vi "GIF.Write.Pack.Data.NormalizeImage__ogtk.vi"(9 "bottom":i16, 10 "right":i16, 11 "ImageIn":u8[](array[numeric])) -> (3 "ImageOut":u8[](array[numeric]))   [LabVIEW 2014]
panel:
  # "GIF.Write.Pack.Data.NormalizeImage.vi\n\nRemoves extra row padding-bytes.\n\nPlease visit http://www.OpenG.org to learn about the\nOpen Source LabVIEW software movement.\n\nNOTICE -- YOU MUST LEAVE THIS NOTICE IN PLACE.  PER THE TERMS OF THE LICENSE BELOW, YOU MAY SUBLICENSE THIS SOFTWARE \nIN ANY WAY THAT DOES NOT CONFLICT WITH THIS LICENSE.\n\n### BSD License (http://www.opensource.org/licenses/bsd-license.php) Begin ###\n \nCopyright (c) 2007, Bill Clench <bclench@yahoo.com>\n\nAll rights reserved.\n\nRedistribution and use in source and binary forms, with or without modification, are permitted provided that the following conditions are met:\n\n    * Redistributions of source code must retain the above copyright notice, this list of conditions and the following disclaimer.\n    * Redistributions in binary form must reproduce the above copyright notice, this list of conditions and the following disclaimer in the \n       documentation and/or other materials provided with the distribution.\n    * Neither the name of SciWare, James Kring, Inc., nor the names of its contributors may be used to endorse or promote products derived \n       from this software without specific prior written permission.\n\nTHIS SOFTWARE IS PROVIDED BY THE COPYRIGHT HOLDERS AND CONTRIBUTORS \"AS IS\" AND ANY EXPRESS OR IMPLIED WARRANTIES, \nINCLUDING, BUT NOT LIMITED TO, THE IMPLIED WARRANTIES OF MERCHANTABILITY AND FITNESS FOR A PARTICULAR PURPOSE ARE \nDISCLAIMED. IN NO EVENT SHALL THE COPYRIGHT OWNER OR CONTRIBUTORS BE LIABLE FOR ANY DIRECT, INDIRECT, INCIDENTAL,\n SPECIAL, EXEMPLARY, OR CONSEQUENTIAL DAMAGES (INCLUDING, BUT NOT LIMITED TO, PROCUREMENT OF SUBSTITUTE GOODS OR \nSERVICES; LOSS OF USE, DATA, OR PROFITS; OR BUSINESS INTERRUPTION) HOWEVER CAUSED AND ON ANY THEORY OF LIABILITY, \nWHETHER IN CONTRACT, STRICT LIABILITY, OR TORT (INCLUDING NEGLIGENCE OR OTHERWISE) ARISING IN ANY WAY OUT OF THE USE \nOF THIS SOFTWARE, EVEN IF ADVISED OF THE POSSIBILITY OF SUCH DAMAGE.\n\n### BSD License End ###"
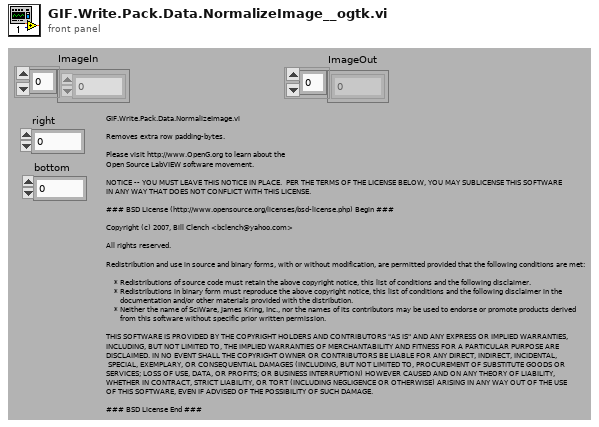
[diagram p1: front panel]
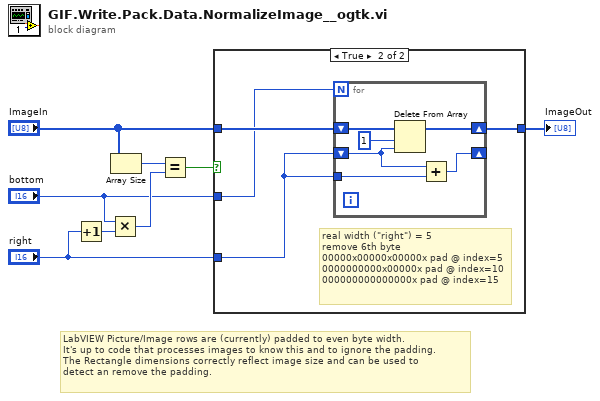
[diagram p0: block diagram]
diagram:
  # "LabVIEW Picture/Image rows are (currently) padded to even byte width.\nIt's up to code that processes images to know this and to ignore the padding.\nThe Rectangle dimensions correctly reflect image size and can be used to\ndetect an remove the padding."
  n1 = Increment(x="right") -> (x+1=w2:i16)
  n2 = Multiply(x="bottom", y=w2) -> (x*y=w7:i16)
  n3 = Array Size(array="ImageIn") -> (size(s)=w8:i32)
  n4 = Equal?(x=w8, y=w7) -> (x = y?=w6:bool)
  n5 = case shown="True" w6 {
    tunnel: "ImageIn" -> [w9 w13]
    tunnel: [w9 w11] -> w4
    tunnel: "right" -> [_ w12]
    tunnel: "bottom" -> [_ w10]
    frame False {
    }
    frame True {
      # "real width (\"right\") = 5\nremove 6th byte\n00000x00000x00000x pad @ index=5\n0000000000x00000x pad @ index=10\n000000000000000x pad @ index=15"
      n6 = for {
        N: w10 -> [_]
        shift-right: [w14] -> w11
        shift-left: w13 -> [w19]
        shift-right: [w15] -> _
        shift-left: w12 -> [w17]
        tunnel: w12 -> [w16]
        n7 = Delete From Array(array=w19, length=1, index=w17) -> (array with subset deleted=w14:u8[])  [unwired: 1 out]
        n8 = Add(x=w17, y=w16) -> (x+y=w15:i16)
      }
    }
  }
  "ImageOut" <- w4
